vi "Read configuration.vi"(8 "error in":errorcluster, 11 "PLTarget cRIO in":refnum<class "PLTarget cRIO.lvclass">) -> (0 "error out":errorcluster, 2 "configuration":refnum<class "NISE_CEF_serializable configuration.lvclass">, 3 "PLTarget cRIO out":refnum<class "PLTarget cRIO.lvclass">)   [LabVIEW 2013, in "PLTarget cRIO.lvclass"]
uses:
  PLTarget cRIO.lvclass
  <vilib>/NI/Configuration Framework/serializable configuration/NISE_CEF_serializable configuration.lvclass
  PLTarget cRIO.lvclass/PLTarget cRIO.ctl
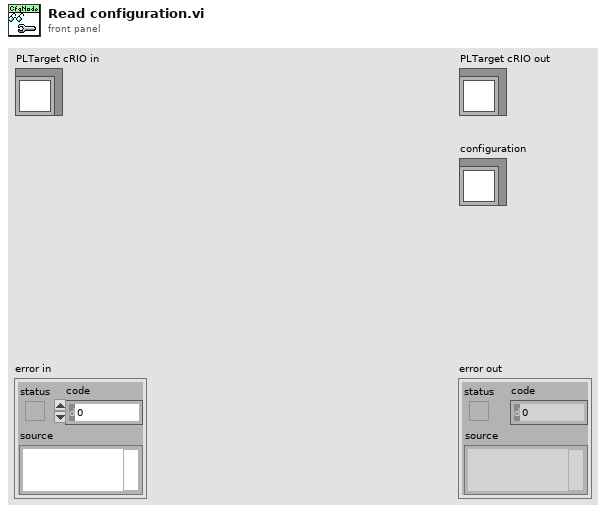
[diagram p1: front panel]
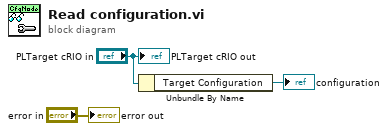
[diagram p0: block diagram]
diagram:
  n1 = Unbundle By Name("PLTarget cRIO in") -> ("Target Configuration"=→"configuration":refnum<class "PL_Target Configuration.lvclass">)
  "error out" <- "error in"
  "PLTarget cRIO out" <- "PLTarget cRIO in"
